vi "List And Filter Controls From VI.vi"(8 "Error In":errorcluster, 11 "VI Refnum":refnum<vi>) -> (0 "Error Out":errorcluster, 3 "Control Lists":T1)   [LabVIEW 2021, in "Appearance Actor.lvlib" / "Appearance Actor.lvclass"]
uses:
  Appearance Actor.lvclass
  Typedefs/Control Reference Lists--cluster.ctl
  Typedefs/Control Reference Lists-TitleBar--cluster.ctl
  Typedefs/Control Reference Lists-SideMenu--cluster.ctl
  Typedefs/Control Reference Lists-BodyPane--cluster.ctl
  Typedefs/Control Reference Lists-StatusBar--cluster.ctl
  <vilib>/regexp/Match Regular Expression.xnode
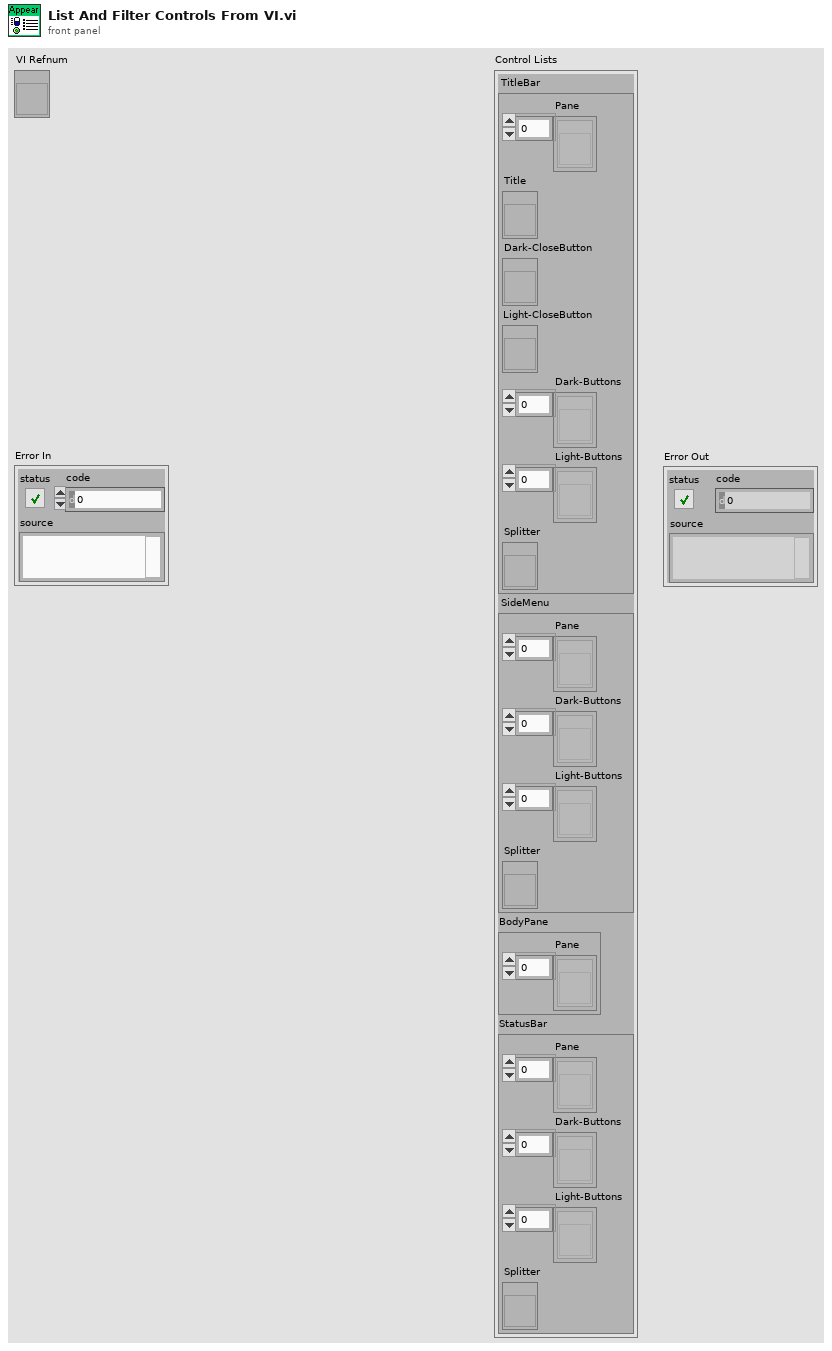
[diagram p1: front panel]
types:
  T1 = typedef "Appearance Actor.lvlib/Appearance Actor.lvclass/Control Reference Lists--cluster.ctl" = cluster{"TitleBar":T2, "SideMenu":T3, "BodyPane":T4, "StatusBar":T5}
  T2 = typedef "Appearance Actor.lvlib/Appearance Actor.lvclass/Control Reference Lists-TitleBar--cluster.ctl" = cluster{"Pane":refnum<vi>[], "Title":refnum<vi>, "Dark-CloseButton":refnum<vi>, "Light-CloseButton":refnum<vi>, "Dark-Buttons":refnum<vi>[], "Light-Buttons":refnum<vi>[], "Splitter":refnum<vi>}
  T3 = typedef "Appearance Actor.lvlib/Appearance Actor.lvclass/Control Reference Lists-SideMenu--cluster.ctl" = cluster{"Pane":refnum<vi>[], "Dark-Buttons":refnum<vi>[], "Light-Buttons":refnum<vi>[], "Splitter":refnum<vi>}
  T4 = typedef "Appearance Actor.lvlib/Appearance Actor.lvclass/Control Reference Lists-BodyPane--cluster.ctl" = cluster{"Pane":refnum<vi>[]}
  T5 = typedef "Appearance Actor.lvlib/Appearance Actor.lvclass/Control Reference Lists-StatusBar--cluster.ctl" = cluster{"Pane":refnum<vi>[], "Dark-Buttons":refnum<vi>[], "Light-Buttons":refnum<vi>[], "Splitter":refnum<vi>}
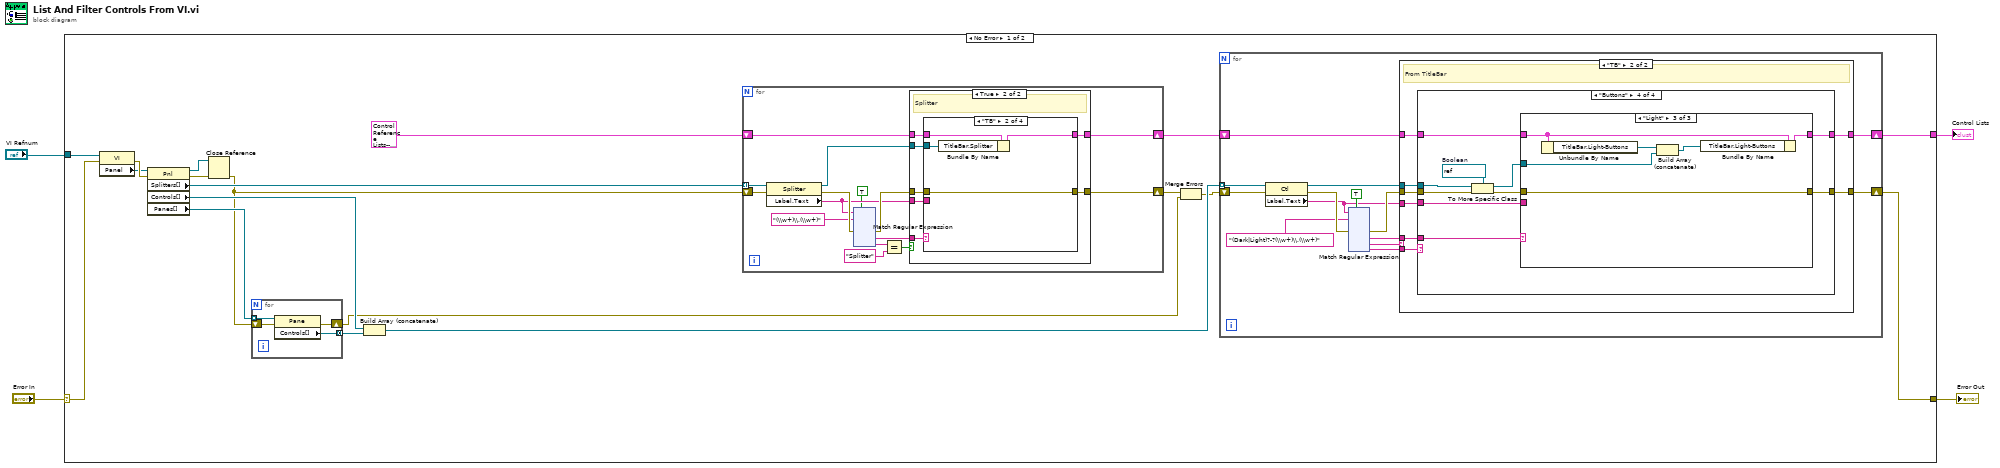
[diagram p0: block diagram]
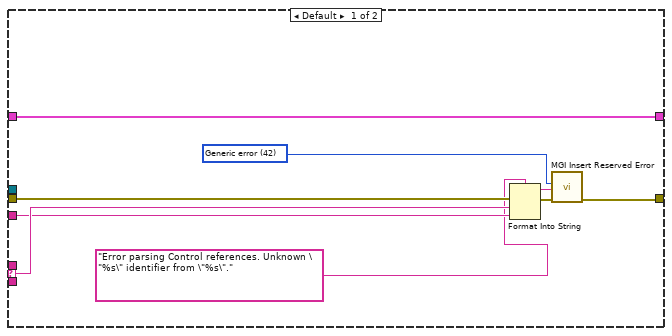
[diagram p2: hidden frame]
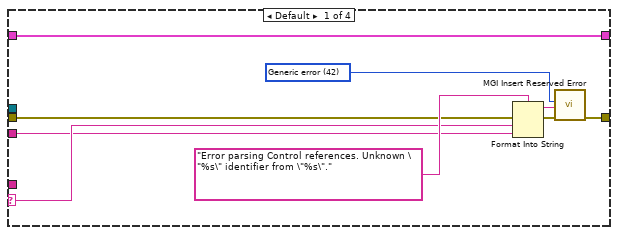
[diagram p3: hidden frame]
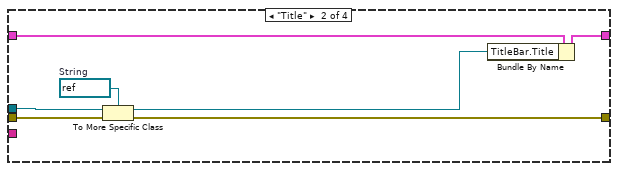
[diagram p4: hidden frame]
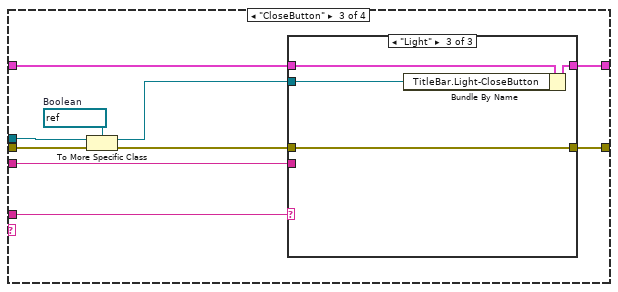
[diagram p5: hidden frame]
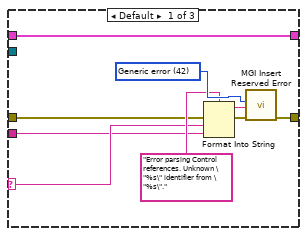
[diagram p6: hidden frame]
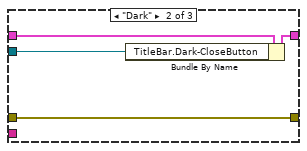
[diagram p7: hidden frame]
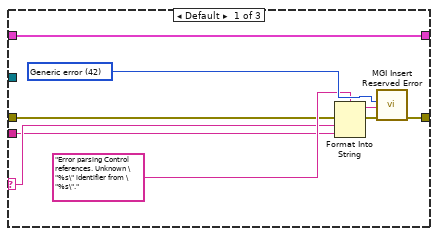
[diagram p8: hidden frame]
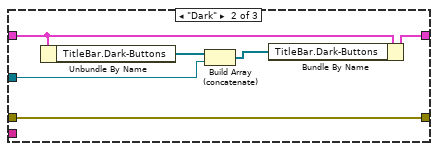
[diagram p9: hidden frame]
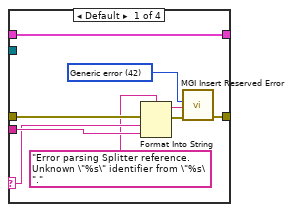
[diagram p11: hidden frame]
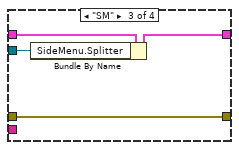
[diagram p12: hidden frame]
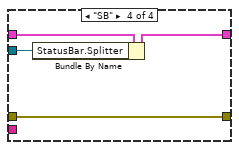
[diagram p13: hidden frame]
diagram:
  n1 = case shown="No Error" "Error In" {
    selector: "Error In" -> [w21 w419]
    tunnel: "VI Refnum" -> [w23 _]
    tunnel: [w8 w419] -> w2
    tunnel: [w7 _] -> w1
    frame No Error {
      n2 = property class="VI"(reference=w23, error in=w21) -> (error out=w20:errorcluster, "Panel"=w19:refnum<vi>)  [unwired: 1 out]
      n3 = property class="Pnl"(reference=w19, error in=w20) -> (reference out=w22:refnum<vi>, error out=w15:errorcluster, "Splitters[]"=w14:refnum<vi>[], "Controls[]"=w17:refnum<vi>[], "Panes[]"=w18:refnum<vi>[])
      n4 = Close Reference(reference=w22, error in (no error)=w15) -> (error out=w13:errorcluster)
      n5 = for {
        tunnel: w18 -> [w418] mode=indexing
        shift-right: [w416] -> w5
        shift-left: w13 -> [w417]
        tunnel: [w415] -> w16 mode=concatenating
        n6 = property class="Pane"(reference=w418, error in=w417) -> (error out=w416:errorcluster, "Controls[]"=w415:refnum<vi>[])  [unwired: 1 out]
      }
      n7 = Build Array (concatenate)(w17, w16) -> (w9:refnum<vi>[])
      n8 = for {
        tunnel: w14 -> [w264] mode=indexing
        shift-right: [w256] -> w10
        shift-left: w13 -> [w263]
        shift-right: [w259] -> w11
        shift-left: T1 {"TitleBar"={"Pane"=[], "Title"=refnum, "Dark-CloseButton"=refnum, "Light-CloseButton"=refnum, "Dark-Buttons"=[], "Light-Buttons"=[], "Splitter"=refnum}, "SideMenu"={"Pane"=[], "Dark-Buttons"=[], "Light-Buttons"=[], "Splitter"=refnum}, "BodyPane"={"Pane"=[]}, "StatusBar"={"Pane"=[], "Dark-Buttons"=[], "Light-Buttons"=[], "Splitter"=refnum}} ("Control Reference Lists") -> [w261]
        n9 = property class="Splitter"(reference=w264, error in=w263) -> (reference out=w258:refnum<vi>, error out=w262:errorcluster, "Label.Text"=w251:string)
        n10 = xnode "Match Regular Expression"("input string"=w251, "regular expression"="(\\w+)\\.(\\w+)", "error in"=w262, "ignore case? (F)"=TRUE) -> ("error out"=w257:errorcluster, "submatch 1"=w260:string, "submatch 2"=w254:string)  [unwired: 2 in, 4 out]
        n11 = Equal?(x=w254, y="Splitter" ("regular expression")) -> (x = y?=w255:bool)
        n12 = case shown="True" w255 {
          tunnel: w261 -> [w265 w273]
          tunnel: w260 -> [_ w272]
          tunnel: [w265 w271] -> w259
          tunnel: w258 -> [_ w270]
          tunnel: w257 -> [w266 w269]
          tunnel: [w266 w268] -> w256
          tunnel: w251 -> [_ w267]
          frame False {
            # "SubSplitter or other"
          }
          frame True {
            # "Splitter"
            n13 = case shown="\"TB\"" w272 {
              selector: w272 -> [w275 _ _ _]
              tunnel: w273 -> [w282 w286 w290 w294]
              tunnel: [w282 w285 w289 w293] -> w271
              tunnel: w270 -> [_ w284 w288 w292]
              tunnel: w269 -> [w278 w283 w287 w291]
              tunnel: [w277 w283 w287 w291] -> w268
              tunnel: w267 -> [w276 _ _ _]
              frame Default {
                w279 = 42 items=["No error", "Argument error", "Memory is full", "Out of zone", "End of file", "File already open", "Generic file I/O error", "File not found", "File permission error", "Disk is full", "Duplicate path", "Too many files open", "System feature not enabled", "Resource file not found", "Cannot add resource", "Resource not found", "Image not found", "Image memory error", "Pen does not exist", "Config type invalid", "Config token not found", "Config parse error", "Config memory error", "Bad external code format", "Bad external code offset", "External code not present", "Null window", "Destroy window error", "Null menu", "Print aborted", "Bad print record", "Print driver error", "Windows error during printing", "Memory error during printing", "Print dialog error", "Generic print error", "Invalid device refnum", "Device not found", "Device parameter error", "Device unit error", "Cannot open device", "Device call aborted", "Generic error", "Cancelled by user", "Object ID too low", "Object ID too high", "Object not in heap", "Unknown heap", "Unknown object (invalid DefProc)", "Unknown object (DefProc not in table)", "Message out of range", "Invalid (null) method", "Unknown message", "Manager call not supported", "Bad address", "Network operation in progress", "Network operation timed out", "Connection is busy", "Network attribute not supported", "Network error", "Address in use", "System out of memory", "Connection aborted", "Connection refused", "Not connected", "Already connected", "Connection closed", "Initialization error (interapplication manager)", "Bad occurrence", "Wait on unbound occurrence handler", "Occurrence queue overflow", "Datalog type conflict", "Unused", "Unrecognized type (interapplication manager)", "Memory corrupt", "Failed to make temporary DLL", "Old CIN version", "Drag socket not found", "Failed to load drop-object", "Failed to register OLE object", "Failed to release OLE object", "Format specifier type mismatch", "Unknown format specifier", "Too few format specifiers", "Too many format specifiers", "Scan failed", "Newer CIN version", "OLE Convert", "Runtime menu error", "Password tampered", "Unknown error code"] ("Reserved Error Code (Generic error)")
                n14 = Format Into String(format string="Error parsing Splitter reference. Unknown \"%s\" identifier from \"%s\".", error in=w278, w275, w276) -> (resulting string=w281:string, error out=w280:errorcluster)  [unwired: 1 in]
                n15 = call <userlib>:"MGI Insert Reserved Error.vi"("Error In"=w280, "Error Description"=w281, "Reserved Error Code (Generic error)"=w279) -> ("Error Out"=w277:errorcluster)  [unwired: 8 in]
              }
              frame "TB" {
                n16 = Bundle By Name(cluster=w286, "TitleBar.Splitter"=w284) -> (w285:T1)
              }
              frame "SM" {
                n17 = Bundle By Name(cluster=w290, "SideMenu.Splitter"=w288) -> (w289:T1)
              }
              frame "SB" {
                n18 = Bundle By Name(cluster=w294, "StatusBar.Splitter"=w292) -> (w293:T1)
              }
            }
          }
        }
      }
      n19 = Merge Errors(w10, w5) -> (w6:errorcluster)
      n20 = for {
        shift-right: [w25] -> w7
        shift-left: w11 -> [w32]
        shift-right: [w30] -> w8
        shift-left: w6 -> [w36]
        tunnel: w9 -> [w37] mode=indexing
        n21 = property class="Ctl"(reference=w37, error in=w36) -> (reference out=w24:refnum<vi>, error out=w35:errorcluster, "Label.Text"=w26:string)
        n22 = xnode "Match Regular Expression"("input string"=w26, "regular expression"="(Dark|Light)?-?(\\w+)\\.(\\w+)", "error in"=w35, "ignore case? (F)"=TRUE) -> ("error out"=w29:errorcluster, "submatch 1"=w28:string, "submatch 2"=w31:string, "submatch 3"=w27:string)  [unwired: 2 in, 4 out]
        n23 = case shown="\"TB\"" w31 {
          selector: w31 -> [w41 _]
          tunnel: w32 -> [w39 w50]
          tunnel: [w42 w52] -> w30
          tunnel: w29 -> [w43 w53]
          tunnel: w28 -> [_ w47]
          tunnel: w27 -> [_ w54]
          tunnel: w26 -> [w40 w51]
          tunnel: [w39 w49] -> w25
          tunnel: w24 -> [_ w48]
          frame Default {
            w44 = 42 items=["No error", "Argument error", "Memory is full", "Out of zone", "End of file", "File already open", "Generic file I/O error", "File not found", "File permission error", "Disk is full", "Duplicate path", "Too many files open", "System feature not enabled", "Resource file not found", "Cannot add resource", "Resource not found", "Image not found", "Image memory error", "Pen does not exist", "Config type invalid", "Config token not found", "Config parse error", "Config memory error", "Bad external code format", "Bad external code offset", "External code not present", "Null window", "Destroy window error", "Null menu", "Print aborted", "Bad print record", "Print driver error", "Windows error during printing", "Memory error during printing", "Print dialog error", "Generic print error", "Invalid device refnum", "Device not found", "Device parameter error", "Device unit error", "Cannot open device", "Device call aborted", "Generic error", "Cancelled by user", "Object ID too low", "Object ID too high", "Object not in heap", "Unknown heap", "Unknown object (invalid DefProc)", "Unknown object (DefProc not in table)", "Message out of range", "Invalid (null) method", "Unknown message", "Manager call not supported", "Bad address", "Network operation in progress", "Network operation timed out", "Connection is busy", "Network attribute not supported", "Network error", "Address in use", "System out of memory", "Connection aborted", "Connection refused", "Not connected", "Already connected", "Connection closed", "Initialization error (interapplication manager)", "Bad occurrence", "Wait on unbound occurrence handler", "Occurrence queue overflow", "Datalog type conflict", "Unused", "Unrecognized type (interapplication manager)", "Memory corrupt", "Failed to make temporary DLL", "Old CIN version", "Drag socket not found", "Failed to load drop-object", "Failed to register OLE object", "Failed to release OLE object", "Format specifier type mismatch", "Unknown format specifier", "Too few format specifiers", "Too many format specifiers", "Scan failed", "Newer CIN version", "OLE Convert", "Runtime menu error", "Password tampered", "Unknown error code"] ("Reserved Error Code (Generic error)")
            n24 = Format Into String(format string="Error parsing Control references. Unknown \"%s\" identifier from \"%s\".", error in=w43, w41, w40) -> (resulting string=w46:string, error out=w45:errorcluster)  [unwired: 1 in]
            n25 = call <userlib>:"MGI Insert Reserved Error.vi"("Error In"=w45, "Error Description"=w46, "Reserved Error Code (Generic error)"=w44) -> ("Error Out"=w42:errorcluster)  [unwired: 8 in]
          }
          frame "TB" {
            # "From TitleBar"
            n26 = case shown="\"Buttons\"" w54 {
              selector: w54 -> [w57 _ _ _]
              tunnel: w53 -> [w59 w65 w75 w102]
              tunnel: [w58 w64 w72 w99] -> w52
              tunnel: w51 -> [w56 _ w71 w98]
              tunnel: w50 -> [w55 w70 w80 w107]
              tunnel: [w55 w69 w79 w106] -> w49
              tunnel: w48 -> [_ w67 w77 w104]
              tunnel: w47 -> [_ _ w74 w101]
              frame Default {
                w61 = 42 items=["No error", "Argument error", "Memory is full", "Out of zone", "End of file", "File already open", "Generic file I/O error", "File not found", "File permission error", "Disk is full", "Duplicate path", "Too many files open", "System feature not enabled", "Resource file not found", "Cannot add resource", "Resource not found", "Image not found", "Image memory error", "Pen does not exist", "Config type invalid", "Config token not found", "Config parse error", "Config memory error", "Bad external code format", "Bad external code offset", "External code not present", "Null window", "Destroy window error", "Null menu", "Print aborted", "Bad print record", "Print driver error", "Windows error during printing", "Memory error during printing", "Print dialog error", "Generic print error", "Invalid device refnum", "Device not found", "Device parameter error", "Device unit error", "Cannot open device", "Device call aborted", "Generic error", "Cancelled by user", "Object ID too low", "Object ID too high", "Object not in heap", "Unknown heap", "Unknown object (invalid DefProc)", "Unknown object (DefProc not in table)", "Message out of range", "Invalid (null) method", "Unknown message", "Manager call not supported", "Bad address", "Network operation in progress", "Network operation timed out", "Connection is busy", "Network attribute not supported", "Network error", "Address in use", "System out of memory", "Connection aborted", "Connection refused", "Not connected", "Already connected", "Connection closed", "Initialization error (interapplication manager)", "Bad occurrence", "Wait on unbound occurrence handler", "Occurrence queue overflow", "Datalog type conflict", "Unused", "Unrecognized type (interapplication manager)", "Memory corrupt", "Failed to make temporary DLL", "Old CIN version", "Drag socket not found", "Failed to load drop-object", "Failed to register OLE object", "Failed to release OLE object", "Format specifier type mismatch", "Unknown format specifier", "Too few format specifiers", "Too many format specifiers", "Scan failed", "Newer CIN version", "OLE Convert", "Runtime menu error", "Password tampered", "Unknown error code"] ("Reserved Error Code (Generic error)")
                n27 = Format Into String(format string="Error parsing Control references. Unknown \"%s\" identifier from \"%s\".", error in=w59, w57, w56) -> (resulting string=w63:string, error out=w62:errorcluster)  [unwired: 1 in]
                n28 = call <userlib>:"MGI Insert Reserved Error.vi"("Error In"=w62, "Error Description"=w63, "Reserved Error Code (Generic error)"=w61) -> ("Error Out"=w58:errorcluster)  [unwired: 8 in]
              }
              frame "Title" {
                w68 = refnum<vi> refnum  # String
                n29 = To More Specific Class(target class=w68, reference=w67, error in=w65) -> (specific class reference=w66:refnum<vi>, error out=w64:errorcluster)
                n30 = Bundle By Name(cluster=w70, "TitleBar.Title"=w66) -> (w69:T1)
              }
              frame "CloseButton" {
                w78 = refnum<vi> refnum  # Boolean
                n31 = To More Specific Class(target class=w78, reference=w77, error in=w75) -> (specific class reference=w76:refnum<vi>, error out=w73:errorcluster)
                n32 = case shown="\"Light\"" w74 {
                  selector: w74 -> [w82 _ _]
                  tunnel: w80 -> [w83 w93 w97]
                  tunnel: [w83 w92 w96] -> w79
                  tunnel: w76 -> [_ w91 w95]
                  tunnel: w73 -> [w85 w90 w94]
                  tunnel: [w84 w90 w94] -> w72
                  tunnel: w71 -> [w81 _ _]
                  frame Default {
                    w87 = 42 items=["No error", "Argument error", "Memory is full", "Out of zone", "End of file", "File already open", "Generic file I/O error", "File not found", "File permission error", "Disk is full", "Duplicate path", "Too many files open", "System feature not enabled", "Resource file not found", "Cannot add resource", "Resource not found", "Image not found", "Image memory error", "Pen does not exist", "Config type invalid", "Config token not found", "Config parse error", "Config memory error", "Bad external code format", "Bad external code offset", "External code not present", "Null window", "Destroy window error", "Null menu", "Print aborted", "Bad print record", "Print driver error", "Windows error during printing", "Memory error during printing", "Print dialog error", "Generic print error", "Invalid device refnum", "Device not found", "Device parameter error", "Device unit error", "Cannot open device", "Device call aborted", "Generic error", "Cancelled by user", "Object ID too low", "Object ID too high", "Object not in heap", "Unknown heap", "Unknown object (invalid DefProc)", "Unknown object (DefProc not in table)", "Message out of range", "Invalid (null) method", "Unknown message", "Manager call not supported", "Bad address", "Network operation in progress", "Network operation timed out", "Connection is busy", "Network attribute not supported", "Network error", "Address in use", "System out of memory", "Connection aborted", "Connection refused", "Not connected", "Already connected", "Connection closed", "Initialization error (interapplication manager)", "Bad occurrence", "Wait on unbound occurrence handler", "Occurrence queue overflow", "Datalog type conflict", "Unused", "Unrecognized type (interapplication manager)", "Memory corrupt", "Failed to make temporary DLL", "Old CIN version", "Drag socket not found", "Failed to load drop-object", "Failed to register OLE object", "Failed to release OLE object", "Format specifier type mismatch", "Unknown format specifier", "Too few format specifiers", "Too many format specifiers", "Scan failed", "Newer CIN version", "OLE Convert", "Runtime menu error", "Password tampered", "Unknown error code"] ("Reserved Error Code (Generic error)")
                    n33 = Format Into String(format string="Error parsing Control references. Unknown \"%s\" identifier from \"%s\".", error in=w85, w82, w81) -> (resulting string=w89:string, error out=w88:errorcluster)  [unwired: 1 in]
                    n34 = call <userlib>:"MGI Insert Reserved Error.vi"("Error In"=w88, "Error Description"=w89, "Reserved Error Code (Generic error)"=w87) -> ("Error Out"=w84:errorcluster)  [unwired: 8 in]
                  }
                  frame "Dark" {
                    n35 = Bundle By Name(cluster=w93, "TitleBar.Dark-CloseButton"=w91) -> (w92:T1)
                  }
                  frame "Light" {
                    n36 = Bundle By Name(cluster=w97, "TitleBar.Light-CloseButton"=w95) -> (w96:T1)
                  }
                }
              }
              frame "Buttons" {
                w105 = refnum<vi> refnum  # Boolean
                n37 = To More Specific Class(target class=w105, reference=w104, error in=w102) -> (specific class reference=w103:refnum<vi>, error out=w100:errorcluster)
                n38 = case shown="\"Light\"" w101 {
                  selector: w101 -> [w109 _ _]
                  tunnel: w107 -> [w110 w120 w126]
                  tunnel: [w110 w122 w128] -> w106
                  tunnel: w103 -> [_ w117 w123]
                  tunnel: w100 -> [w112 w121 w127]
                  tunnel: [w111 w121 w127] -> w99
                  tunnel: w98 -> [w108 _ _]
                  frame Default {
                    w114 = 42 items=["No error", "Argument error", "Memory is full", "Out of zone", "End of file", "File already open", "Generic file I/O error", "File not found", "File permission error", "Disk is full", "Duplicate path", "Too many files open", "System feature not enabled", "Resource file not found", "Cannot add resource", "Resource not found", "Image not found", "Image memory error", "Pen does not exist", "Config type invalid", "Config token not found", "Config parse error", "Config memory error", "Bad external code format", "Bad external code offset", "External code not present", "Null window", "Destroy window error", "Null menu", "Print aborted", "Bad print record", "Print driver error", "Windows error during printing", "Memory error during printing", "Print dialog error", "Generic print error", "Invalid device refnum", "Device not found", "Device parameter error", "Device unit error", "Cannot open device", "Device call aborted", "Generic error", "Cancelled by user", "Object ID too low", "Object ID too high", "Object not in heap", "Unknown heap", "Unknown object (invalid DefProc)", "Unknown object (DefProc not in table)", "Message out of range", "Invalid (null) method", "Unknown message", "Manager call not supported", "Bad address", "Network operation in progress", "Network operation timed out", "Connection is busy", "Network attribute not supported", "Network error", "Address in use", "System out of memory", "Connection aborted", "Connection refused", "Not connected", "Already connected", "Connection closed", "Initialization error (interapplication manager)", "Bad occurrence", "Wait on unbound occurrence handler", "Occurrence queue overflow", "Datalog type conflict", "Unused", "Unrecognized type (interapplication manager)", "Memory corrupt", "Failed to make temporary DLL", "Old CIN version", "Drag socket not found", "Failed to load drop-object", "Failed to register OLE object", "Failed to release OLE object", "Format specifier type mismatch", "Unknown format specifier", "Too few format specifiers", "Too many format specifiers", "Scan failed", "Newer CIN version", "OLE Convert", "Runtime menu error", "Password tampered", "Unknown error code"] ("Reserved Error Code (Generic error)")
                    n39 = Format Into String(format string="Error parsing Control references. Unknown \"%s\" identifier from \"%s\".", error in=w112, w109, w108) -> (resulting string=w116:string, error out=w115:errorcluster)  [unwired: 1 in]
                    n40 = call <userlib>:"MGI Insert Reserved Error.vi"("Error In"=w115, "Error Description"=w116, "Reserved Error Code (Generic error)"=w114) -> ("Error Out"=w111:errorcluster)  [unwired: 8 in]
                  }
                  frame "Dark" {
                    n41 = Unbundle By Name(w120) -> ("TitleBar.Dark-Buttons"=w119:refnum<vi>[])
                    n42 = Build Array (concatenate)(w119, w117) -> (w118:refnum<vi>[])
                    n43 = Bundle By Name(cluster=w120, "TitleBar.Dark-Buttons"=w118) -> (w122:T1)
                  }
                  frame "Light" {
                    n44 = Unbundle By Name(w126) -> ("TitleBar.Light-Buttons"=w125:refnum<vi>[])
                    n45 = Build Array (concatenate)(w125, w123) -> (w124:refnum<vi>[])
                    n46 = Bundle By Name(cluster=w126, "TitleBar.Light-Buttons"=w124) -> (w128:T1)
                  }
                }
              }
            }
          }
        }
      }
    }
    frame Error {
    }
  }
  "Error Out" <- w2
  "Control Lists" <- w1
